vi "to_global_coords.vi"(8 "error in":errorcluster, 9 "orientation":cluster{"pitch":dbl, "roll":dbl, "yaw":dbl}, 10 "offset":cluster{"x":dbl, "y":dbl, "z":dbl}, 11 "local":cluster{"x":dbl, "y":dbl, "z":dbl}) -> (0 "error out":errorcluster, 3 "global":cluster{"x":dbl, "y":dbl, "z":dbl})   [LabVIEW 2011, in "gVision.lvlib"]
uses:
  gVision.lvlib
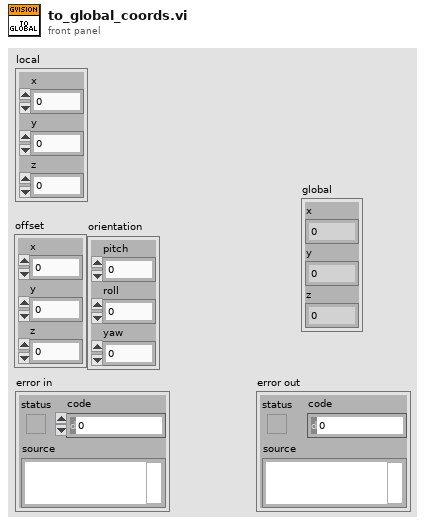
[diagram p1: front panel]
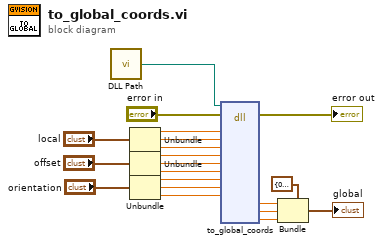
[diagram p0: block diagram]
diagram:
  n1 = call "DLL Path.vi"() -> ("DLL Path"=w20:path)  [unwired: 5 in]
  n2 = Unbundle("local") -> ("x"=w16:dbl, "y"=w15:dbl, "z"=w14:dbl)
  n3 = Unbundle("offset") -> ("x"=w12:dbl, "y"=w11:dbl, "z"=w10:dbl)
  n4 = Unbundle("orientation") -> ("pitch"=w8:dbl, "roll"=w7:dbl, "yaw"=w6:dbl)
  n5 = dll-call lib="?" fn="to_global_coords"(path in=w20, error in="error in", "local_x"=w16, "local_y"=w15, "local_z"=w14, "offset_x"=w12, "offset_y"=w11, "offset_z"=w10, "pitch"=w8, "roll"=w7, "yaw"=w6) -> (error out=→"error out":errorcluster, "global_x"=w4:dbl, "global_y"=w3:dbl, "global_z"=w2:dbl)  [unwired: 14 in, 1 out]
  n6 = Bundle(cluster=cluster{"x":dbl, "y":dbl, "z":dbl} {"x"=0.0, "y"=0.0, "z"=0.0} ("local 2"), "x"=w4, "y"=w3, "z"=w2) -> (→"global":cluster{"x":dbl, "y":dbl, "z":dbl})
